vi "OCV_4309_ApertureTime_StdDev.vi"() -> ()   [LabVIEW 2019]
panel:
  out "Aperture Time (s)":dbl[](array[numeric]) format="%#_6p"
  in  "Sample Rates (Hz)":dbl[](array[numeric])=[10.0, 12.0, 15.0, 20.0, 30.0, 60.0, 100.0, 200.0, 500.0, 1000.0, 5000.0, 10000.0]
  in  "Std Dev (V)":dbl[](array[numeric])=[4.912673562937666e-07, 5.511090249899113e-07, 4.905858067345527e-07, 4.784668974350132e-07, 5.558108956489086e-07, 8.069426585679406e-07, 6.99075825748838e-07, 2.7921160159506675e-06, 0.0002740086748828484, 1.8338541503295823e-06, 3.640955207646567e-06, 6.986958822834755e-06] format="%#_6p"
  in  "Range (V)":dbl[](array[numeric])=[2.127932607676186e-06, 2.440394776925814e-06, 2.113632086020445e-06, 2.292495077771406e-06, 2.3593223847928613e-06, 3.074985451601009e-06, 3.0511786610620817e-06, 1.0014437655803121e-05, 0.0006255797503784688, 8.165792197312172e-06, 1.4182235513970909e-05, 2.6380023109728867e-05] format="%#_6p"
  in  "Elapsed Time (ms)":u32[](array[numeric])=[7049, 6034, 4984, 3900, 2850, 1785, 1370, 1049, 1051, 1050, 852, 826]
  in  "Test Time (s)":dbl[](array[numeric])=[1.467, 1.478, 1.811, 2.23, 3.314, 4.35, 5.415, 6.481, 7.55] format="%#_6p"
  in  "Range (V)":dbl[](array[numeric])=[1.7445e-05, 4.778e-06, 4.275e-06, 3.342e-06, 2.417e-06, 2.021e-06, 1.994e-06, 1.792e-06, 1.572e-06] format="%#_6p"
  in  "Standard Deviation (V)":dbl[](array[numeric])=[4.767e-06, 1.2e-06, 9.26045e-07, 8.04748e-07, 5.57873e-07, 4.88194e-07, 4.82016e-07, 4.21724e-07, 3.65671e-07] format="%#_6p"
  in  "4309 Aperture Time (s)":dbl[](array[numeric])=[0.002, 0.005, 0.01, 0.0166666, 0.033333, 0.05, 0.0666666, 0.0833333, 0.1] format="%#_6p"
  out "4309 Standard Deviation vs Aperture Time":T1(graph)={"Standard Deviation (Ohm)"=[0.002, 0.005, 0.01, 0.0166666, 0.033333, 0.05, 0.0666666, 0.0833333, 0.1], "Aperture Time (s)"=[4.767e-06, 1.2e-06, 9.26045e-07, 8.04748e-07, 5.57873e-07, 4.88194e-07, 4.82016e-07, 4.21724e-07, 3.65671e-07]}
  # "128 channels"
  # "500 Hz"
  # "200 Hz"
  # "100 Hz"
  # "60 Hz"
  # "30 Hz"
  # "20 Hz"
  # "15 Hz"
  # "12 Hz"
  # "10 Hz"
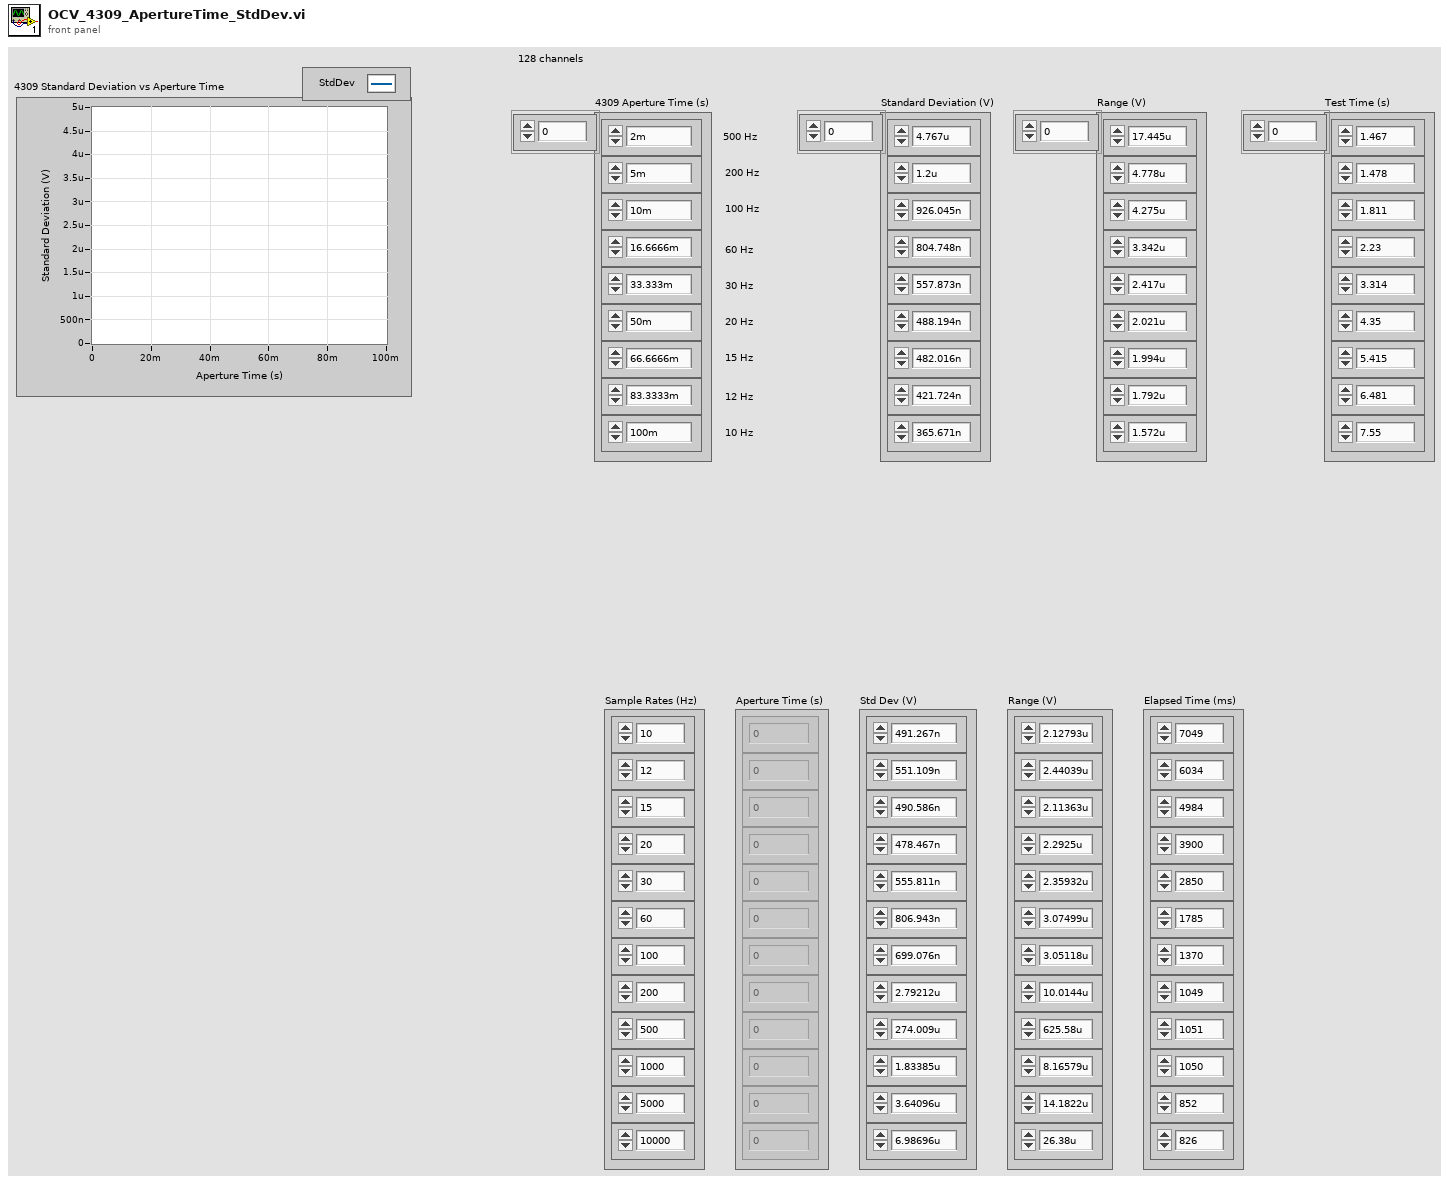
[diagram p1: front panel]
types:
  T1 = cluster{"Standard Deviation (Ohm)":dbl[], "Aperture Time (s)":dbl[]}
  T2 = cluster{"4309 Aperture Time (s)":dbl[], "Standard Deviation (V)":dbl[]}
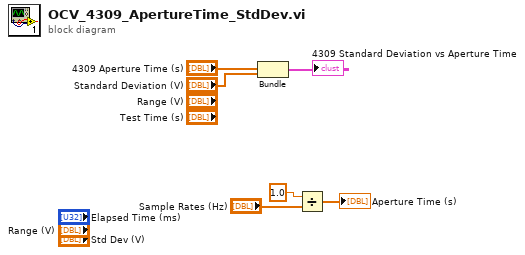
[diagram p0: block diagram]
diagram:
  n1 = Bundle("4309 Aperture Time (s)"="4309 Aperture Time (s)", "Standard Deviation (V)"="Standard Deviation (V)") -> (→"4309 Standard Deviation vs Aperture Time":T2)  [unwired: 1 in]
  n2 = Divide(x=1.0, y="Sample Rates (Hz)") -> (x/y=→"Aperture Time (s)":dbl[])
